vi "RT fast measure v1.1.vi"() -> ()   [LabVIEW 2023]
uses:
  RT fast data.ctl
  <vilib>/LabVIEW Targets/FPGA/cRIO/shared/nicrio_ModuleControls/nicrio_cRIO-9775_RecordDataRates4ChansRing.ctl
  <vilib>/FPGAPlugInAG/cRIO-9063/niLvFpga_Open_cRIO-9063.vi
  <vilib>/rvi/interface/common/dynamic/niFpgaDynamicAddResources.vi
  <vilib>/FPGAPlugInAG/Dynamic/niLvFpga_Reset_Dynamic.vi
  <vilib>/Utility/error.llb/Error Cluster From Error Code.vi
  <vilib>/rvi/errors/niLvFpgaAdjustHostInterfaceError.vi
  <vilib>/FPGAPlugInAG/Dynamic/niLvFpga_Run_Dynamic.vi
  <vilib>/RVI Host/nirviSupport.llb/nirviErrorClusterFromErrorCode.vi
  <vilib>/FPGAPlugInAG/Dynamic/niLvFpga_Close_Dynamic.vi
  <vilib>/rvi/interface/nirviOpenFPGA/nirviOpenFPGA.xnode
  Transport measurement/FPGA Bitfiles/Mainproject_FPGATarget_Icreadoutclocked_PcJtOPDfEmI.lvbitx
  Ic readout_clocked_delayed trigger_dist V3.1.vi
  <vilib>/rvi/interface/nirviMethod/nirviMethod.xnode
  <vilib>/rvi/interface/nirviReadWriteControl/nirviReadWriteControl.xnode
  <vilib>/rvi/interface/nirviCloseFPGA/nirviCloseFPGA.xnode
  <resource>/objmgr/ni.dex.rc
  <vilib>/rvi/interface/nirviMethod/StockFPGA_InlinedMethodWaitForSingleIRQ.vi
  <vilib>/FPGAPlugInAG/Dynamic/niLvFpga_WaitOnIrq_Dynamic.vi
  <vilib>/FPGAPlugInAG/Dynamic/niLvFpga_AcknowledgeIrq_Dynamic.vi
  <vilib>/FPGAPlugInAG/Dynamic/niLvFpga_ReadFifo_Dynamic.vi
  <vilib>/rvi/errors/niLvFpgaMergeErrorWithErrorCode.vi
  NiFpgaLv.dll
  <vilib>/rvi/interface/Simulation/niFpgaSimulationCallBeginRW.vi
panel:
  out "error out":errorcluster
  in  "Parameters":T1={"Records Num"=10000, "AI Trigger Configuration"={"Trigger Slope"=enum."Positive", "Trigger Level"=0.1298828125, "Hystesis Value"=0.0, "AI Channel"=0}, "Record PreTrigger Samples"=1, "Record Samples"=16, "Ic Cut off or curve"=TRUE, "Gate wait time us"=150, "Record Data Rate"=1, "Count us half of T"=15000, "Wait before trigger us"=10100, "Cutoff delay usec"=0} {"Record Data Rate" items=["20.000 MS/s (NI 9775)"=1, "10.00 MS/s (NI 9775)"=2, "6.667 MS/s (NI 9775)"=3, "5.000 MS/s (NI 9775)"=4, "2.500 MS/s (NI 9775)"=8, "1.667 MS/s (NI 9775)"=12, "1.250 MS/s (NI 9775)"=16, "1.000 MS/s (NI 9775)"=20, "833.333 KS/s (NI 9775)"=24, "714.286 KS/s (NI 9775)"=28, "625.000 KS/s (NI 9775)"=32, "555.556 KS/s (NI 9775)"=36, "500.000 KS/s (NI 9775)"=40, "454.545 KS/s (NI 9775)"=44, "416.667 KS/s (NI 9775)"=48, "384.615 KS/s (NI 9775)"=52, "357.143 KS/s (NI 9775)"=56, "333.333 KS/s (NI 9775)"=60, "312.500 KS/s (NI 9775)"=64, "294.118 KS/s (NI 9775)"=68, "277.778 KS/s (NI 9775)"=72, "263.158 KS/s (NI 9775)"=76, "250.000 KS/s (NI 9775)"=80, "238.095 KS/s (NI 9775)"=84, "227.273 KS/s (NI 9775)"=88, "217.391 KS/s (NI 9775)"=92, "208.333 KS/s (NI 9775)"=96, "200.000 KS/s (NI 9775)"=100, "192.308 KS/s (NI 9775)"=104, "185.185 KS/s (NI 9775)"=108, "178.571 KS/s (NI 9775)"=112, "172.414 KS/s (NI 9775)"=116, "166.667 KS/s (NI 9775)"=120, "161.290 KS/s (NI 9775)"=124, "156.250 KS/s (NI 9775)"=128, "151.515 KS/s (NI 9775)"=132, "147.059 KS/s (NI 9775)"=136, "142.857 KS/s (NI 9775)"=140, "138.889 KS/s (NI 9775)"=144, "135.135 KS/s (NI 9775)"=148, "131.579 KS/s (NI 9775)"=152, "128.205 KS/s (NI 9775)"=156, "125.000 KS/s (NI 9775)"=160, "121.951 KS/s (NI 9775)"=164, "119.048 KS/s (NI 9775)"=168, "116.279 KS/s (NI 9775)"=172, "113.636 KS/s (NI 9775)"=176, "111.111 KS/s (NI 9775)"=180, "108.696 KS/s (NI 9775)"=184, "106.383 KS/s (NI 9775)"=188, "104.167 KS/s (NI 9775)"=192, "102.041 KS/s (NI 9775)"=196, "100.000 KS/s (NI 9775)"=200, "50.000 KS/s (NI 9775)"=400, "33.333 KS/s (NI 9775)"=600, "25.000 KS/s (NI 9775)"=800, "20.000 KS/s (NI 9775)"=1000, "16.667 KS/s (NI 9775)"=1200, "14.286 KS/s (NI 9775)"=1400, "12.500 KS/s (NI 9775)"=1600, "11.111 KS/s (NI 9775)"=1800, "10.000 KS/s (NI 9775)"=2000, "9.091 KS/s (NI 9775)"=2200, "8.333 KS/s (NI 9775)"=2400, "7.692 KS/s (NI 9775)"=2600, "7.143 KS/s (NI 9775)"=2800, "6.667 KS/s (NI 9775)"=3000, "6.250 KS/s (NI 9775)"=3200, "5.882 KS/s (NI 9775)"=3400, "5.556 KS/s (NI 9775)"=3600, "5.000 KS/s (NI 9775)"=4000, "4.762 KS/s (NI 9775)"=4200, "4.545 KS/s (NI 9775)"=4400, "4.348 KS/s (NI 9775)"=4600, "4.167 KS/s (NI 9775)"=4800, "4.000 KS/s (NI 9775)"=5000, "3.846 KS/s (NI 9775)"=5200, "3.571 KS/s (NI 9775)"=5600, "3.333 KS/s (NI 9775)"=6000, "3.125 KS/s (NI 9775)"=6400, "2.941 KS/s (NI 9775)"=6800, "2.778 KS/s (NI 9775)"=7200, "2.632 KS/s (NI 9775)"=7600, "2.500 KS/s (NI 9775)"=8000, "2.381 KS/s (NI 9775)"=8400, "2.273 KS/s (NI 9775)"=8800, "2.174 KS/s (NI 9775)"=9200, "2.083 KS/s (NI 9775)"=9600, "2.000 KS/s (NI 9775)"=10000, "1.923 KS/s (NI 9775)"=10400, "1.852 KS/s (NI 9775)"=10800, "1.786 KS/s (NI 9775)"=11200, "1.724 KS/s (NI 9775)"=11600, "1.667 KS/s (NI 9775)"=12000, "1.613 KS/s (NI 9775)"=12400, "1.563 KS/s (NI 9775)"=12800, "1.515 KS/s (NI 9775)"=13200, "1.471 KS/s (NI 9775)"=13600, "1.429 KS/s (NI 9775)"=14000, "1.389 KS/s (NI 9775)"=14400, "1.351 KS/s (NI 9775)"=14800, "1.316 KS/s (NI 9775)"=15200, "1.282 KS/s (NI 9775)"=15600, "1.250 KS/s (NI 9775)"=16000, "1.220 KS/s (NI 9775)"=16400, "1.190 KS/s (NI 9775)"=16800, "1.163 KS/s (NI 9775)"=17200, "1.136 KS/s (NI 9775)"=17600, "1.111 KS/s (NI 9775)"=18000, "1.087 KS/s (NI 9775)"=18400, "1.064 KS/s (NI 9775)"=18800, "1.042 KS/s (NI 9775)"=19200, "1.020 KS/s (NI 9775)"=19600, "1.000 KS/s (NI 9775)"=20000, "0.980 KS/s (NI 9775)"=20400, "0.962 KS/s (NI 9775)"=20800, "0.943 KS/s (NI 9775)"=21200, "0.926 KS/s (NI 9775)"=21600, "0.909 KS/s (NI 9775)"=22000, "0.893 KS/s (NI 9775)"=22400, "0.877 KS/s (NI 9775)"=22800, "0.862 KS/s (NI 9775)"=23200, "0.847 KS/s (NI 9775)"=23600, "0.833 KS/s (NI 9775)"=24000, "0.820 KS/s (NI 9775)"=24400, "0.806 KS/s (NI 9775)"=24800, "0.794 KS/s (NI 9775)"=25200, "0.781 KS/s (NI 9775)"=25600, "0.694 KS/s (NI 9775)"=28800, "0.625 KS/s (NI 9775)"=32000, "0.568 KS/s (NI 9775)"=35200, "0.521 KS/s (NI 9775)"=38400, "0.446 KS/s (NI 9775)"=44800, "0.391 KS/s (NI 9775)"=51200, "0.347 KS/s (NI 9775)"=57600, "0.313 KS/s (NI 9775)"=64000]}
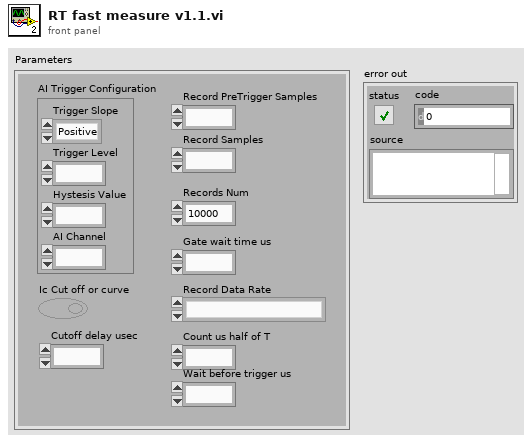
[diagram p1: front panel]
types:
  T1 = typedef "RT fast data.ctl" = cluster{"Records Num":i32, "AI Trigger Configuration":cluster{"Trigger Slope":enum8{"Positive", "Negative"}, "Trigger Level":fxp<+/-,17,5>, "Hystesis Value":fxp<+,16,4>, "AI Channel":u8}, "Record PreTrigger Samples":u32, "Record Samples":u32, "Ic Cut off or curve":bool, "Gate wait time us":u32, "Record Data Rate":T2, "Count us half of T":u32, "Wait before trigger us":u32, "Cutoff delay usec":u32}
  T2 = typedef "nicrio_cRIO-9775_RecordDataRates4ChansRing.ctl" = u16
  T3 = cluster{"Trigger Slope":enum8{"Positive", "Negative"}, "Trigger Level":fxp<+/-,17,5>, "Hystesis Value":fxp<+,16,4>, "AI Channel":u8}
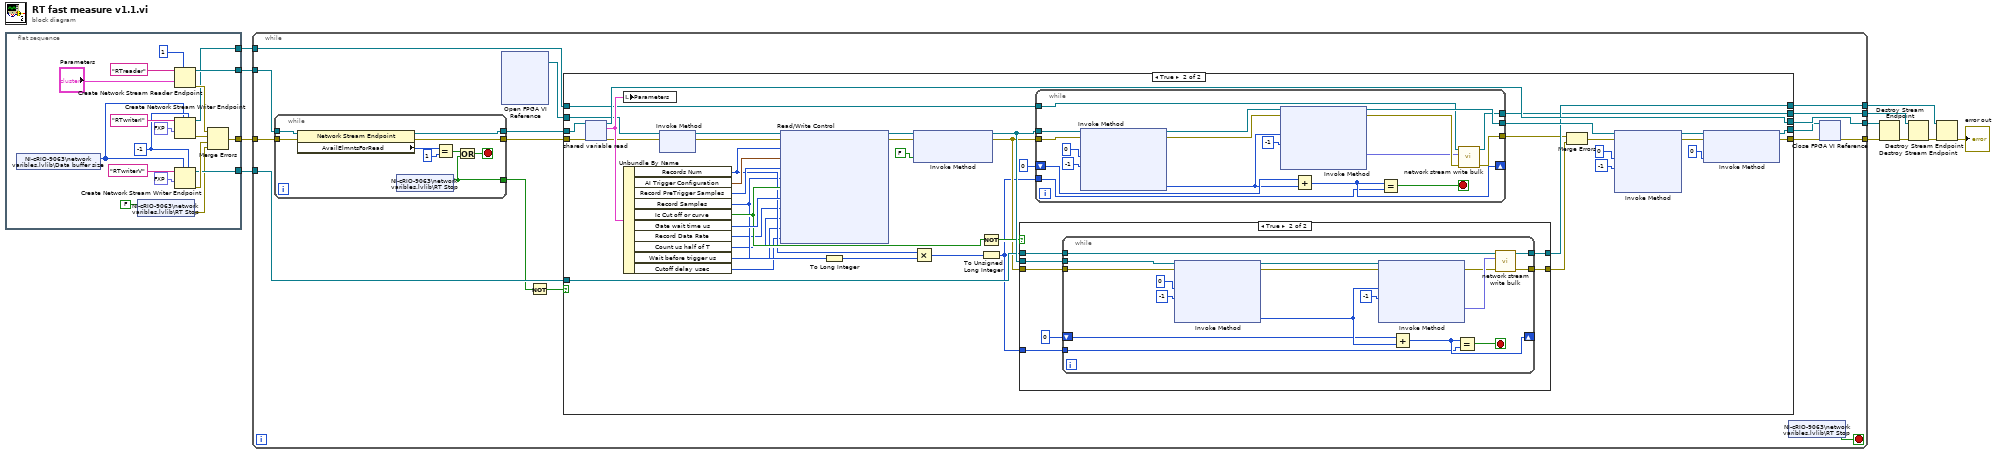
[diagram p0: block diagram]
diagram:
  n1 = flat-sequence {
    tunnel: [w27] -> w11
    tunnel: [w17] -> w10
    tunnel: [w16] -> w5
    tunnel: [w15] -> w4
    frame #0 {
      w22 = -1 ("timeout in ms (-1)")
      n2 = shared-variable "NI-cRIO-9063\\network varibles.lvlib\\Data buffer size"() -> (w21:i32)  [unwired: 1 in, 1 out]
      n3 = shared-variable "NI-cRIO-9063\\network varibles.lvlib\\RT Stop"(FALSE ("RT Stop")) -> (error out=w13:errorcluster)  [unwired: 1 in]
      n4 = Create Network Stream Reader Endpoint(7:1 ("reader buffer size"), 9:"Parameters", 11:"RTreader" ("reader name")) -> (0:w20:errorcluster, 3:w27:refnum<k21>)  [unwired: 4 in]
      n5 = Create Network Stream Writer Endpoint(5:w22, 7:w21, 9:fxp<+/-,17,5> 0.0, 11:"RTwriterI" ("writer name")) -> (0:w19:errorcluster, 3:w16:refnum<k21>)  [unwired: 3 in]
      n6 = Create Network Stream Writer Endpoint(5:w22, 7:w21, 9:fxp<+/-,17,5> 0.0, 11:"RTwriterV" ("writer name")) -> (0:w18:errorcluster, 3:w15:refnum<k21>)  [unwired: 3 in]
      n7 = Merge Errors(w20, w19, w18, w13) -> (w17:errorcluster)
    }
  }
  n8 = while {
    tunnel: w11 -> [w45]
    tunnel: w10 -> [w44]
    tunnel: [w31] -> w1
    tunnel: [w41] -> w9
    tunnel: w5 -> [w37]
    tunnel: w4 -> [w36]
    tunnel: [w35] -> w3
    tunnel: [w34] -> w2
    stop <- w40 stop-if-true
    n9 = while {
      tunnel: w45 -> [w146]
      tunnel: w44 -> [w145]
      tunnel: [w144] -> w43
      tunnel: [w143] -> w42
      tunnel: [w138] -> w30
      stop <- w139 stop-if-true
      n10 = property class="Network Stream Endpoint"(reference=w146, error in=w145) -> (reference out=w144:refnum<k21>, error out=w143:errorcluster, "AvailElmntsForRead"=w142:i32)
      n11 = shared-variable "NI-cRIO-9063\\network varibles.lvlib\\RT Stop"() -> (w138:bool)  [unwired: 1 in, 1 out]
      n12 = Equal?(x=w142, y=1) -> (x = y?=w140:bool)
      n13 = Or(x=w140, y=w138) -> (x .or. y?=w139:bool)
    }
    n14 = xnode "Open FPGA VI Reference"() -> ("FPGA VI Reference Out"=w38:refnum<k20>)  [unwired: 2 in, 1 out]
    n15 = Not(x=w30) -> (.not. x?=w39:bool)
    n16 = case shown="True" w39 {
      tunnel: w43 -> [w49 w88]
      tunnel: w42 -> [w50 w53]
      tunnel: [w48 w79] -> w33
      tunnel: [w50 w78] -> w32
      tunnel: [w49 w77] -> w41
      tunnel: w38 -> [w48 w54]
      tunnel: w37 -> [w47 w64]
      tunnel: w36 -> [w46 w66]
      tunnel: [w47 w63] -> w35
      tunnel: [w46 w65] -> w34
      frame False {
      }
      frame True {
        n17 = shared-variable-read(w88, w53) -> (w77:refnum<k21>, w52:errorcluster, w87:T1)  [unwired: 1 in, 1 out]
        n18 = local write "Parameters"(w87) -> ()
        n19 = Unbundle By Name(w87) -> ("Records Num"=w70:i32, "AI Trigger Configuration"=w90:T3, "Record PreTrigger Samples"=w89:u32, "Record Samples"=w69:u32, "Ic Cut off or curve"=w73:bool, "Gate wait time us"=w86:u32, "Record Data Rate"=w61:T2, "Count us half of T"=w56:u32, "Wait before trigger us"=w55:u32, "Cutoff delay usec"=w51:u32)
        n20 = xnode "Invoke Method"("FPGA VI Reference In"=w54, "error in"=w52) -> ("FPGA VI Reference Out"=w92:refnum<k20>, "error out"=w71:errorcluster)
        n21 = xnode "Read/Write Control"("FPGA VI Reference In"=w92, "error in"=w71, "Records Num"=w70, "AI Trigger Configuration"=w90, "Record PreTrigger Samples"=w89, "Record Samples"=w69, "Ic Cut off or curve"=w73, "Gate wait time us"=w86, "Record Data Rate"=w61, "Count us"=w56, "Wait before trigger us"=w55, "Cutoff delay usec"=w51) -> ("FPGA VI Reference Out"=w93:refnum<k20>, "error out"=w57:errorcluster)
        n22 = To Long Integer(number=w69) -> (32bit integer=w68:i32)
        n23 = xnode "Invoke Method"("FPGA VI Reference In"=w93, "error in"=w57, "Wait Until Done (F)"=FALSE) -> ("FPGA VI Reference Out"=w76:refnum<k20>, "error out"=w59:errorcluster)
        n24 = Multiply(x=w70, y=w68) -> (x*y=w67:i32)
        n25 = Not(x=w73) -> (.not. x?=w72:bool)
        n26 = To Unsigned Long Integer(number=w67) -> (unsigned 32bit integer=w58:u32)
        n27 = case shown="True" w72 {
          tunnel: w76 -> [_ w120]
          tunnel: [w112 w114] -> w75
          tunnel: w66 -> [w113 w119]
          tunnel: [w113 w115] -> w65
          tunnel: w59 -> [w112 w117]
          tunnel: w58 -> [_ w116]
          frame False {
          }
          frame True {
            n28 = while {
              tunnel: w120 -> [w130]
              tunnel: w119 -> [w125]
              shift-right: [w127] -> _
              shift-left: u32 0 ("Number of Elements") -> [w129]
              tunnel: w117 -> [w128]
              tunnel: w116 -> [w126]
              tunnel: [w124] -> w115
              tunnel: [w121] -> w114
              stop <- w131 stop-if-true
              n29 = xnode "Invoke Method"("FPGA VI Reference In"=w130, "error in"=w128, "Number of Elements"=u32 0, "Timeout (ms)"=-1) -> ("FPGA VI Reference Out"=w135:refnum<k20>, "error out"=w136:errorcluster, "Elements Remaining"=w137:u32)  [unwired: 1 out]
              n30 = xnode "Invoke Method"("FPGA VI Reference In"=w135, "error in"=w136, "Number of Elements"=w137, "Timeout (ms)"=-1) -> ("error out"=w122:errorcluster, "Data"=w123:fxp<+/-,17,5>[])  [unwired: 2 out]
              n31 = Add(x=w129, y=w137) -> (x+y=w127:u32)
              n32 = Equal?(x=w127, y=w126) -> (x = y?=w131:bool)
              n33 = call "network stream write bulk.vi"("error in (no error)"=w122, "Data"=w123, "endpoint in"=w125) -> ("error out"=w121:errorcluster, "endpoint out"=w124:refnum<k21>)  [unwired: 7 in]
            }
          }
        }
        n34 = while {
          tunnel: w64 -> [w95]
          tunnel: [w96] -> w63
          tunnel: w76 -> [w109]
          tunnel: [w110] -> w85
          tunnel: w59 -> [w107]
          tunnel: [w97] -> w62
          shift-right: [w101] -> _
          shift-left: u32 0 ("Number of Elements") -> [w103]
          tunnel: w58 -> [w100]
          stop <- w99 stop-if-true
          n35 = xnode "Invoke Method"("FPGA VI Reference In"=w109, "error in"=w107, "Number of Elements"=u32 0, "Timeout (ms)"=-1) -> ("FPGA VI Reference Out"=w108:refnum<k20>, "error out"=w106:errorcluster, "Elements Remaining"=w102:u32)  [unwired: 1 out]
          n36 = xnode "Invoke Method"("FPGA VI Reference In"=w108, "error in"=w106, "Number of Elements"=w102, "Timeout (ms)"=-1) -> ("FPGA VI Reference Out"=w110:refnum<k20>, "error out"=w98:errorcluster, "Data"=w94:fxp<+/-,17,5>[])  [unwired: 1 out]
          n37 = Add(x=w103, y=w102) -> (x+y=w101:u32)
          n38 = Equal?(x=w101, y=w100) -> (x = y?=w99:bool)
          n39 = call "network stream write bulk.vi"("error in (no error)"=w98, "Data"=w94, "endpoint in"=w95) -> ("error out"=w97:errorcluster, "endpoint out"=w96:refnum<k21>)  [unwired: 7 in]
        }
        n40 = Merge Errors(w62, w75) -> (w74:errorcluster)
        n41 = xnode "Invoke Method"("FPGA VI Reference In"=w85, "error in"=w74, "IRQ Number(s)"=0, "Timeout (ms)"=-1) -> ("FPGA VI Reference Out"=w82:refnum<k20>, "error out"=w81:errorcluster)  [unwired: 2 out]
        n42 = xnode "Invoke Method"("FPGA VI Reference In"=w82, "error in"=w81, "IRQ Number(s)"=0) -> ("FPGA VI Reference Out"=w79:refnum<k20>, "error out"=w78:errorcluster)
      }
    }
    n43 = shared-variable "NI-cRIO-9063\\network varibles.lvlib\\RT Stop"() -> (w40:bool)  [unwired: 1 in, 1 out]
    n44 = xnode "Close FPGA VI Reference"("FPGA VI Reference In"=w33, "error in"=w32) -> ("error out"=w31:errorcluster)
  }
  n45 = Destroy Stream Endpoint(8:w1, 11:w9) -> (0:w8:errorcluster)
  n46 = Destroy Stream Endpoint(8:w8, 11:w3) -> (0:w7:errorcluster)
  n47 = Destroy Stream Endpoint(8:w7, 11:w2) -> (0:→"error out":errorcluster)
